vi "Dynamic Load DAQmx.vi"(8 "Error In":errorcluster) -> (0 "Error Out":errorcluster, 1 "Synthesizers Out":refnum<class "Pulse Driver.lvclass">[](array[class]), 2 "Device names":string[](array[string]), 3 "Digitizers out":refnum<class "Pulse Driver.lvclass">[](array[class]))   [LabVIEW 2021]
uses:
  Instruments/Pulse Driver/Pulse Driver.lvclass
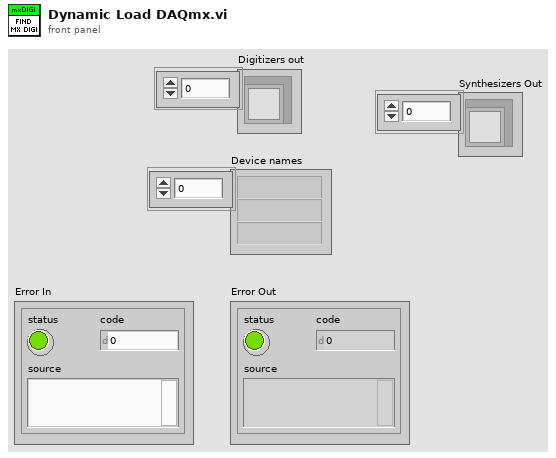
[diagram p1: front panel]
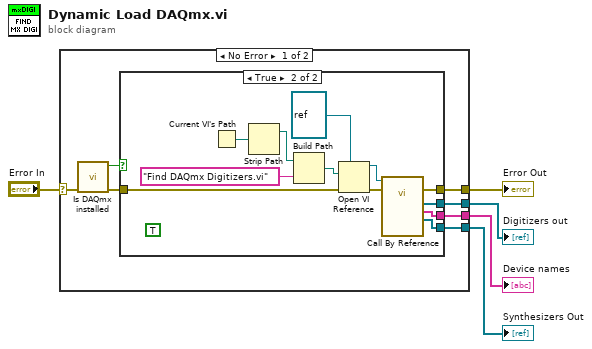
[diagram p0: block diagram]
diagram:
  n1 = case shown="No Error" "Error In" {
    selector: "Error In" -> [w10 w26]
    tunnel: [w12 w26] -> w3
    tunnel: [w8 _] -> w5
    tunnel: [w7 _] -> w4
    tunnel: [w6 _] -> w1
    frame No Error {
      n2 = call "Is DAQmx installed.vi"("Error In"=w10) -> ("Error Out"=w9:errorcluster, "file or folder exists?"=w11:bool)  [unwired: 9 in]
      n3 = case shown="True" w11 {
        tunnel: w9 -> [w13 w20]
        tunnel: [w13 w17] -> w12
        tunnel: [_ w18] -> w8
        tunnel: [_ w15] -> w7
        tunnel: [_ w14] -> w6
        frame False {
        }
        frame True {
          (unwired) TRUE ("DAQmx loaded")
          n4 = Current VI's Path() -> (path=w24:path)
          n5 = Strip Path(path=w24) -> (stripped path=w16:path)  [unwired: 1 out]
          n6 = Build Path(base path=w16, name or relative path="Find DAQmx Digitizers.vi") -> (appended path=w19:path)
          n7 = Open VI Reference(type specifier VI Refnum (for type only)=refnum<vi> refnum, vi path=w19, error in (no error)=w20) -> (vi reference=w22:refnum<vi>, error out=w21:errorcluster)  [unwired: 3 in]
          n8 = call-by-ref "?"(reference=w22, error in=w21) -> (error out=w17:errorcluster, "Synthesizers Out"=w14:refnum<class "Pulse Driver.lvclass">[], "Device names"=w18:string[], "Digitizers out"=w15:refnum<class "Pulse Driver.lvclass">[])  [unwired: 8 in, 2 out]
        }
      }
    }
    frame Error {
    }
  }
  "Error Out" <- w3
  "Digitizers out" <- w4
  "Device names" <- w5
  "Synthesizers Out" <- w1
